vi "Excel_Save.vi"(7 "report file path":path, 8 "error in (no error)":errorcluster, 9 "password (\"\")":string, 10 "prompt to replace? (F)":bool, 11 "Excel._Workbook":refnum<k7>) -> (0 "error out":errorcluster)   [LabVIEW 2015]
doc: "自己改的Excel报表的保存"
uses:
  <vilib>/addons/_office/NI_ReportGenerationToolkit.lvlib
  <vilib>/Utility/NIReport.llb/NI_ReportGenerationCore.lvlib
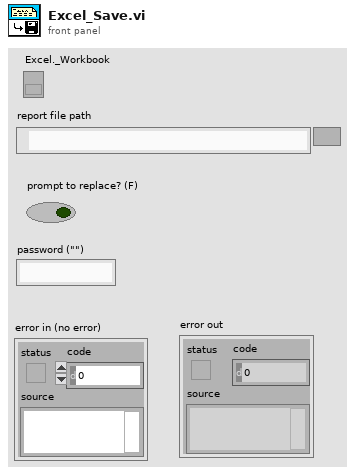
[diagram p1: front panel]
types:
  T1 = enum16{"open", "replace", "create", "open or create", "replace or create", "replace or create with confirmation"}
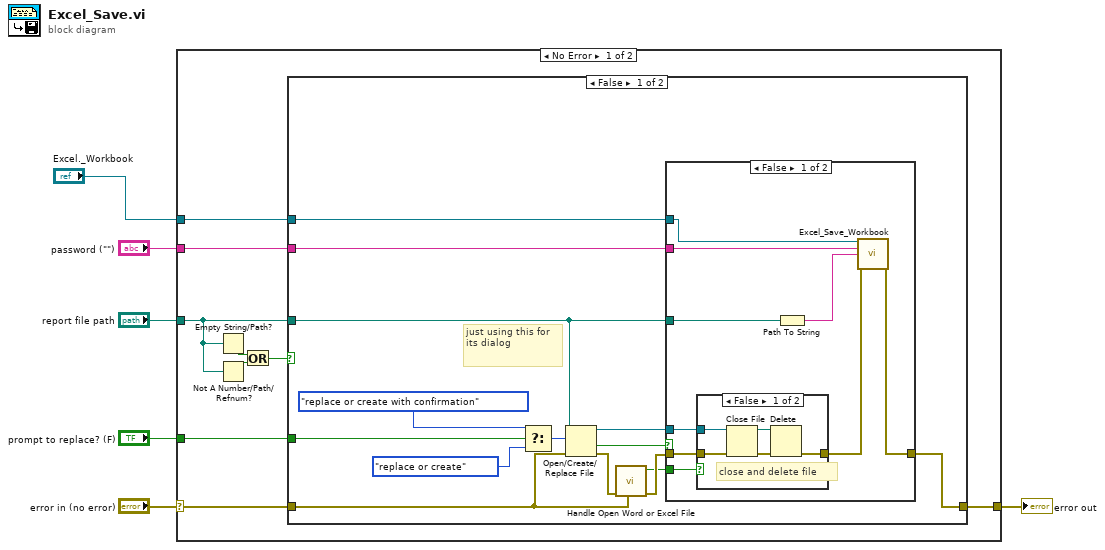
[diagram p0: block diagram]
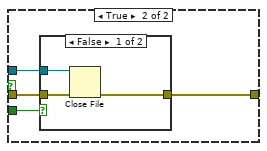
[diagram p3: hidden frame]
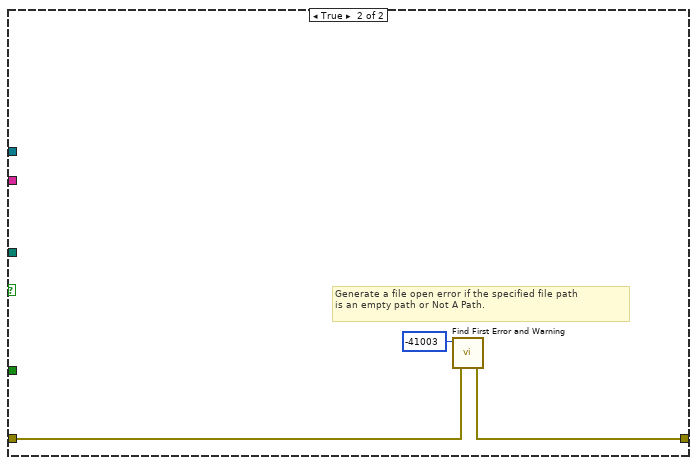
[diagram p5: hidden frame]
diagram:
  n1 = case shown="No Error" "error in (no error)" {
    selector: "error in (no error)" -> [w11 w56]
    tunnel: "report file path" -> [w12 _]
    tunnel: [w10 w56] -> w4
    tunnel: "password (\"\")" -> [w9 _]
    tunnel: "prompt to replace? (F)" -> [w8 _]
    tunnel: "Excel._Workbook" -> [w7 _]
    frame No Error {
      n2 = Empty String/Path?(string/path=w12) -> (empty?=w14:bool)
      n3 = Not A Number/Path/Refnum?(number/path/refnum=w12) -> (NaN/Path/Refnum?=w13:bool)
      n4 = Or(x=w14, y=w13) -> (x .or. y?=w15:bool)
      n5 = case shown="False" w15 {
        tunnel: w12 -> [w19 _]
        tunnel: w11 -> [w20 w54]
        tunnel: [w24 w53] -> w10
        tunnel: w9 -> [w29 _]
        tunnel: w8 -> [w21 _]
        tunnel: w7 -> [w16 _]
        frame False {
          # "just using this for its dialog"
          n6 = Select(t=T1."replace or create with confirmation" ("operation (0:open)"), s=w21, f=T1."replace or create" ("operation (0:open)")) -> (s? t:f=w28:T1)
          n7 = Open/Create/Replace File(file path (use dialog)=w19, error in=w20, operation (0:open)=w28) -> (refnum out=w25:refnum<file>, cancelled=w18:bool, error out=w23:errorcluster)  [unwired: 3 out]
          n8 = call <vilib>:"Handle Open Word or Excel File.vi"("previous error"=w20, "file error"=w23) -> ("error out"=w22:errorcluster, "Error 5 or 6?"=w17:bool)  [unwired: 3 in, 5 out]
          n9 = case shown="False" w18 {
            tunnel: w19 -> [w37 _]
            tunnel: w29 -> [w36 _]
            tunnel: w22 -> [w34 w47]
            tunnel: w25 -> [w35 w48]
            tunnel: [w32 w46] -> w24
            tunnel: w17 -> [w31 w45]
            tunnel: w16 -> [w30 _]
            frame False {
              n10 = case shown="False" w31 {
                tunnel: w35 -> [w41 _]
                tunnel: w34 -> [w40 w44]
                tunnel: [w39 w44] -> w33
                frame False {
                  # "close and delete file"
                  n11 = Close File(refnum=w41, error in=w40) -> (path=w42:path, error out=w43:errorcluster)
                  n12 = Delete(path (use dialog)=w42, error in=w43) -> (error out=w39:errorcluster)  [unwired: 5 out]
                }
                frame True {
                }
              }
              n13 = Path To String(path=w37) -> (string=w38:string)
              n14 = call <vilib>:"Excel_Save_Workbook.vi"("Excel._Workbook"=w30, "password"=w36, "path"=w38, "error in (no error)"=w33) -> ("error out"=w32:errorcluster)  [unwired: 1 in, 10 out]
            }
            frame True {
              n15 = case shown="False" w45 {
                tunnel: w48 -> [w51 _]
                tunnel: w47 -> [w50 w52]
                tunnel: [w49 w52] -> w46
                frame False {
                  n16 = Close File(refnum=w51, error in=w50) -> (error out=w49:errorcluster)  [unwired: 1 out]
                }
                frame True {
                }
              }
            }
          }
        }
        frame True {
          # "Generate a file open error if the specified file path\nis an empty path or Not A Path."
          n17 = call <vilib>:"Find First Error and Warning.vi"("error in (no error)"=w54, "error code"=-41003) -> ("error out"=w53:errorcluster)  [unwired: 1 in, 4 out]
        }
      }
    }
    frame Error {
    }
  }
  "error out" <- w4
